vi "Set Initialize Create Test Node.vi"(8 "error in (no error)":errorcluster, 10 "Initialize Create Test Node":bool, 11 "Abstract Initialize Create Test Node Msg in":refnum<class "Abstract Initialize Create Test Node Msg.lvclass">) -> (0 "error out":errorcluster, 3 "Abstract Initialize Create Test Node Msg out":refnum<class "Abstract Initialize Create Test Node Msg.lvclass">)   [LabVIEW 2013, in "Create Test Node Model.lvlib" / "Abstract Initialize Create Test Node Msg.lvclass"]
uses:
  Abstract Initialize Create Test Node Msg.lvclass
  Abstract Initialize Create Test Node Msg.lvclass/Abstract Initialize Create Test Node Msg.ctl
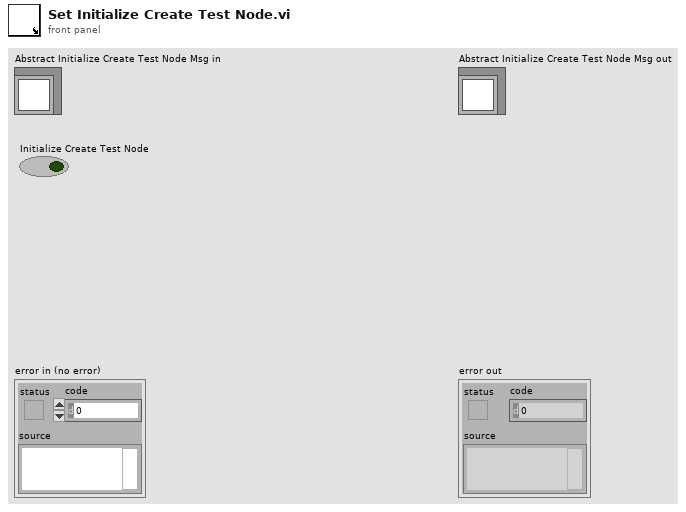
[diagram p1: front panel]
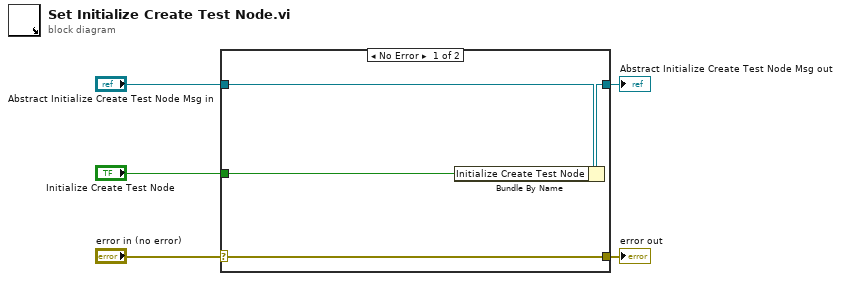
[diagram p0: block diagram]
diagram:
  n1 = case shown="No Error" "error in (no error)" {
    selector: "error in (no error)" -> [w9 w10]
    tunnel: [w9 w10] -> w4
    tunnel: [w7 w11] -> w2
    tunnel: "Abstract Initialize Create Test Node Msg in" -> [w8 w11]
    tunnel: "Initialize Create Test Node" -> [w6 _]
    frame No Error {
      n2 = Bundle By Name(cluster=w8, "Initialize Create Test Node"=w6) -> (w7:refnum<class "Abstract Initialize Create Test Node Msg.lvclass">)
    }
    frame Error {
    }
  }
  "error out" <- w4
  "Abstract Initialize Create Test Node Msg out" <- w2
